vi "Check Piece VS Wall Positions.vi"(8 "Error In":errorcluster caption="Entrée d'erreur", 10 "Piece Coordinates":T1[](array[typedef]), 11 "Brick Wall":T1[](array[typedef])) -> (0 "Error Out":errorcluster caption="Sortie d'erreur", 3 "Invalid Move":bool)   [LabVIEW 2017]
uses:
  Controls/Coordinates.ctl
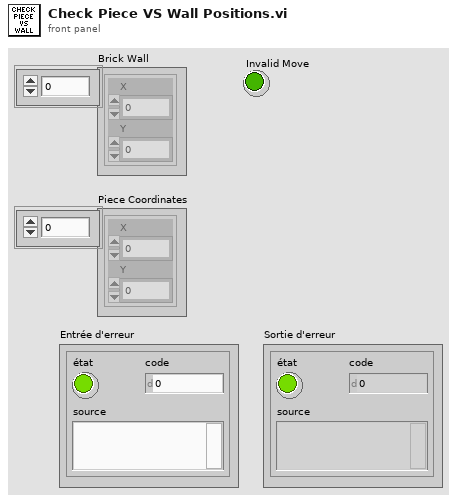
[diagram p1: front panel]
types:
  T1 = typedef "Coordinates.ctl" = cluster{"X":i32, "Y":i32}
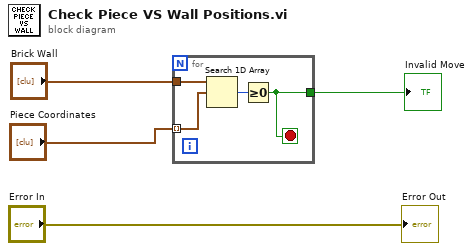
[diagram p0: block diagram]
diagram:
  n1 = for {
    tunnel: "Brick Wall" -> [w8]
    tunnel: "Piece Coordinates" -> [w7] mode=indexing
    tunnel: [w5] -> w3
    stop <- w5 stop-if-true
    n2 = Search 1D Array(1D array=w8, element=w7) -> (index of element=w6:i32)  [unwired: 1 in]
    n3 = Greater Or Equal To 0?(x=w6) -> (x >= 0?=w5:bool)
  }
  "Invalid Move" <- w3
  "Error Out" <- "Error In"
